vi "builder_options.vi"(8 "error in (no error)":errorcluster, 9 "path_index":i32, 10 "configuration":string, 11 "json.provider in":refnum<class "json.provider.lvclass">) -> (0 "error out":errorcluster, 3 "json.provider out":refnum<class "json.provider.lvclass">)   [LabVIEW 2021, in "json.provider.lvclass"]
uses:
  json.provider.lvclass
  json_provider_options.ctl
  json.provider.lvclass/json.provider.ctl
  <vilib>/Utility/sysdir.llb/System Directory Type.ctl
panel:
  # "Default behavior is no options loaded."
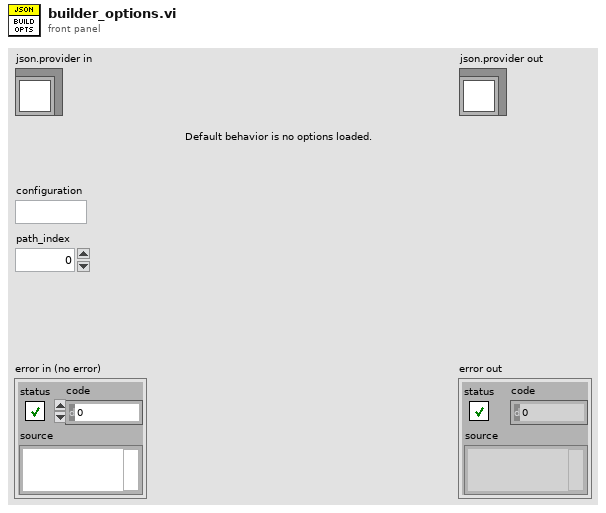
[diagram p1: front panel]
types:
  T1 = enum16{"open", "replace", "create", "open or create", "replace or create", "replace or create with confirmation"}
  T2 = typedef "json.provider.lvclass/json_provider_options.ctl" = cluster{"path":string}
  T3 = typedef "System Directory Type.ctl" = i32
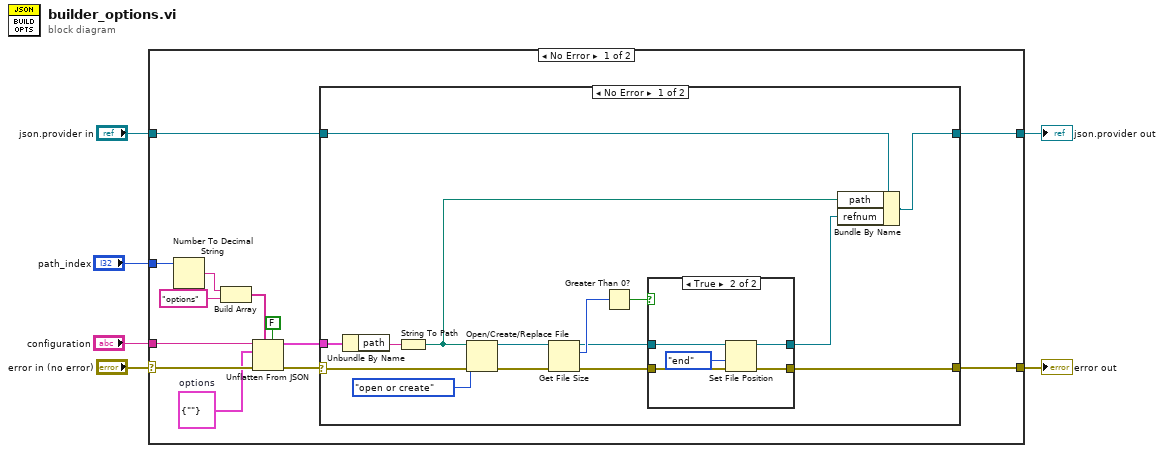
[diagram p0: block diagram]
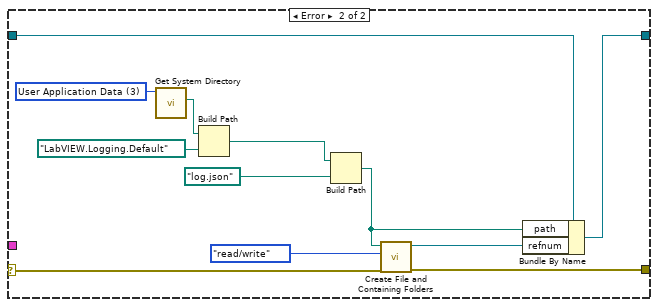
[diagram p3: hidden frame]
diagram:
  n1 = case shown="No Error" "error in (no error)" {
    selector: "error in (no error)" -> [w16 w54]
    tunnel: "json.provider in" -> [w17 w55]
    tunnel: [w19 w55] -> w4
    tunnel: [w18 w54] -> w3
    tunnel: "path_index" -> [w15 _]
    tunnel: "configuration" -> [w13 _]
    frame No Error {
      w10 = T2 {"path"=""}  # options
      n2 = Number To Decimal String(number=w15) -> (decimal integer string=w14:string)  [unwired: 1 in]
      n3 = Build Array(w14, "options" ("element")) -> (w11:string[])
      n4 = Unflatten From JSON(path=w11, enable LabVIEW extensions? (T)=FALSE, JSON string=w13, type and defaults=w10, error in (no error)=w16) -> (value=w7:T2, error out=w8:errorcluster)  [unwired: 2 in]
      n5 = case shown="No Error" w8 {
        selector: w8 -> [w29 w42]
        tunnel: w17 -> [w33 w48]
        tunnel: [w32 w44] -> w19
        tunnel: [w20 w43] -> w18
        tunnel: w7 -> [w30 _]
        frame No Error {
          n6 = Unbundle By Name(w30) -> ("path"=w34:string)
          n7 = String To Path(string=w34) -> (path=w31:path)
          n8 = Open/Create/Replace File(file path (use dialog)=w31, error in=w29, operation (0:open)=T1."open or create") -> (refnum out=w26:refnum<file>, error out=w27:errorcluster)  [unwired: 3 in, 1 out]
          n9 = Get File Size(file=w26, error in=w27) -> (refnum out=w23:refnum<file>, size (in bytes)=w25:i64, 0:w22:errorcluster)
          n10 = Greater Than 0?(x=w25) -> (x > 0?=w24:bool)
          n11 = case shown="True" w24 {
            tunnel: w23 -> [w36 w40]
            tunnel: w22 -> [w35 w39]
            tunnel: [w35 w38] -> w20
            tunnel: [w36 w37] -> w21
            frame False {
            }
            frame True {
              n12 = Set File Position(refnum=w40, from (0:start)=enum16{"start", "end", "current"}."end", error in=w39) -> (refnum out=w37:refnum<file>, error out=w38:errorcluster)  [unwired: 1 in]
            }
          }
          n13 = Bundle By Name(cluster=w33, "path"=w31, "refnum"=w21) -> (w32:refnum<class "json.provider.lvclass">)
        }
        frame Error {
          w53 = T3 3 items=["User Home"=0, "User Desktop"=1, "User Documents"=2, "User Application Data"=3, "User Preferences"=4, "User Temporary"=5, "Public Documents"=6, "Public Application Data"=7, "Public Preferences"=8, "Public Cache"=13, "System Core Libraries"=9, "System Installed Libraries"=10, "Application Files"=11, "Boot Volume Root"=12] ("system directory type")
          n14 = call <vilib>:"Get System Directory.vi"("system directory type"=w53) -> ("system directory"=w52:path)  [unwired: 10 in]
          n15 = Build Path(base path=w52, name or relative path=path "LabVIEW.Logging.Default") -> (appended path=w50:path)
          n16 = Build Path(base path=w50, name or relative path=path "log.json") -> (appended path=w45:path)
          n17 = call <vilib>:"Create File and Containing Folders.vi"("error in (no error)"=w42, "access"=enum16{"read/write", "read-only", "write-only"}."read/write", "file path"=w45) -> ("error out"=w43:errorcluster, "refnum out"=w47:refnum<file>)  [unwired: 7 in]
          n18 = Bundle By Name(cluster=w48, "path"=w45, "refnum"=w47) -> (w44:refnum<class "json.provider.lvclass">)
        }
      }
    }
    frame Error {
    }
  }
  "error out" <- w3
  "json.provider out" <- w4
